vi "PusherSetPosition.vi"(10 "index":i32) -> ()   [LabVIEW 2014, in "PusherLib.lvlib"]
uses:
  PusherLib.lvlib
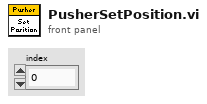
[diagram p1: front panel]
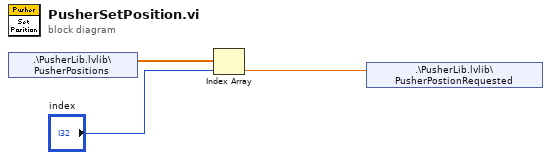
[diagram p0: block diagram]
diagram:
  n1 = shared-variable ".\\PusherLib.lvlib\\PusherPositions"() -> (w3:dbl[])  [unwired: 1 in, 1 out]
  n2 = Index Array(array=w3, index="index") -> (element=w1:dbl)
  n3 = shared-variable ".\\PusherLib.lvlib\\PusherPostionRequested"(w1) -> ()  [unwired: 1 in, 1 out]
